vi "Uim900Recv wrapper.vi"(7 "len":i32, 8 "error in (no error)":errorcluster caption="错误输入（无错误）", 9 "pRcvDate":string, 10 "dwCanNodeId":u32, 11 "dwDevIndex":u32) -> (0 "error out":errorcluster caption="错误输出", 1 "pRcvDate out":string, 3 "function return":u32)   [LabVIEW 2016, in "UISimCanFunc_wrapper.lvlib"]
doc: "_declspec (dllexport) DWORD Uim900Recv_wrapper(DWORD dwDevIndex, DWORD dwCanNodeId, char pRcvDate[], int len);"
uses:
  <userlib>/UISimCanFunc_wrapper/UISimCanFunc_wrapper.lvlib
  <userlib>/UISimCanFunc_wrapper/UISimCanFunc_wrapper.dll
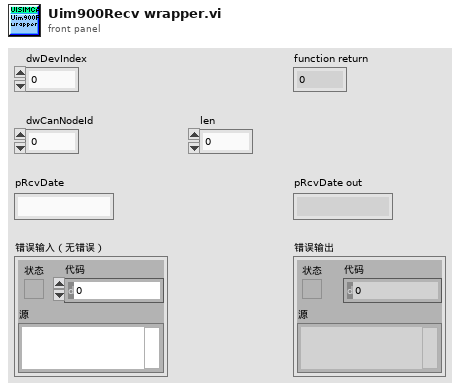
[diagram p1: front panel]
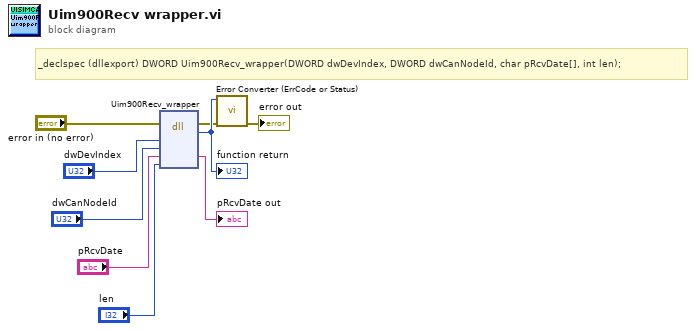
[diagram p0: block diagram]
diagram:
  # "_declspec (dllexport) DWORD Uim900Recv_wrapper(DWORD dwDevIndex, DWORD dwCanNodeId, char pRcvDate[], int len);"
  n1 = dll-call lib="C:/Program Files (x86)/National Instruments/LabVIEW 2016/user.lib/UISimCanFunc_wrapper/UISimCanFunc_wrapper.*" fn="Uim900Recv_wrapper"(error in="error in (no error)", "dwDevIndex"="dwDevIndex", "dwCanNodeId"="dwCanNodeId", "pRcvDate"="pRcvDate", "len"="len") -> (error out=w2:errorcluster, w9:u32, "pRcvDate"=→"pRcvDate out":string)  [unwired: 5 in, 1 out]
  "function return" <- w9
  n2 = call <userlib>:"Error Converter (ErrCode or Status).vi"("error in (no error)"=w2, "error code"=w9) -> ("error out"=→"error out":errorcluster)  [unwired: 9 in]
